vi "EditorPopUp.vi"(8 "error in (no error)":errorcluster, 11 "MAUI.Editor":refnum<class "MAUI.Editor.lvclass">) -> (0 "error out":errorcluster, 3 "MAUI.Editor out":refnum<class "MAUI.Editor.lvclass">)   [LabVIEW 2020, in "MAUI.Editor.lvclass"]
uses:
  MAUI.Editor/MAUI.Editor.lvclass
panel:
  in  "Listbox":i32(listbox)
  in  "Save":bool
  in  "Select":bool
  in  "Refresh":bool
  in  "Configure":bool
  in  "New":bool
  in  "Delete":bool
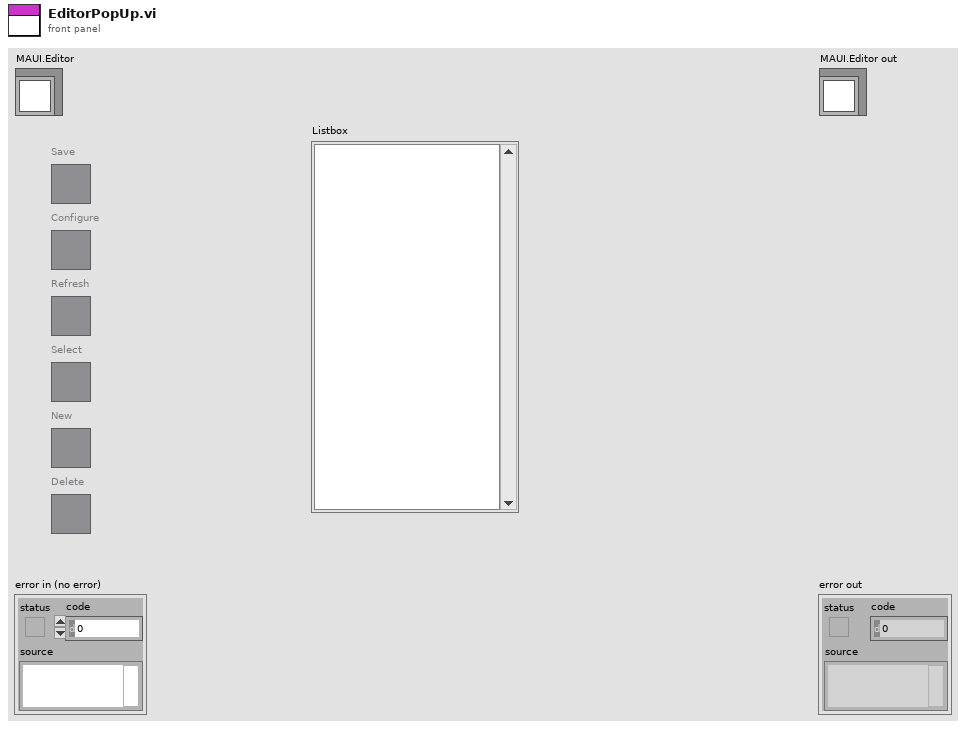
[diagram p1: front panel]
types:
  T1 = enum32{"Invalid", "Standard", "Closed", "Hidden", "Minimized", "Maximized"}
  T2 = enum32{"invalid app kind", "Development System", "Run Time System", "Student Edition", "Embedded LabVIEW", "Evaluation", "Custom"}
  T3 = cluster{"Core":cluster{"Current VI Reference":refnum<vi>, "Close Panel on Exit?":bool}, "MAUI.Editor":refnum<class "MAUI.Editor.lvclass">}
  T4 = cluster{"Current VI Reference":refnum<vi>, "Close Panel on Exit?":bool}
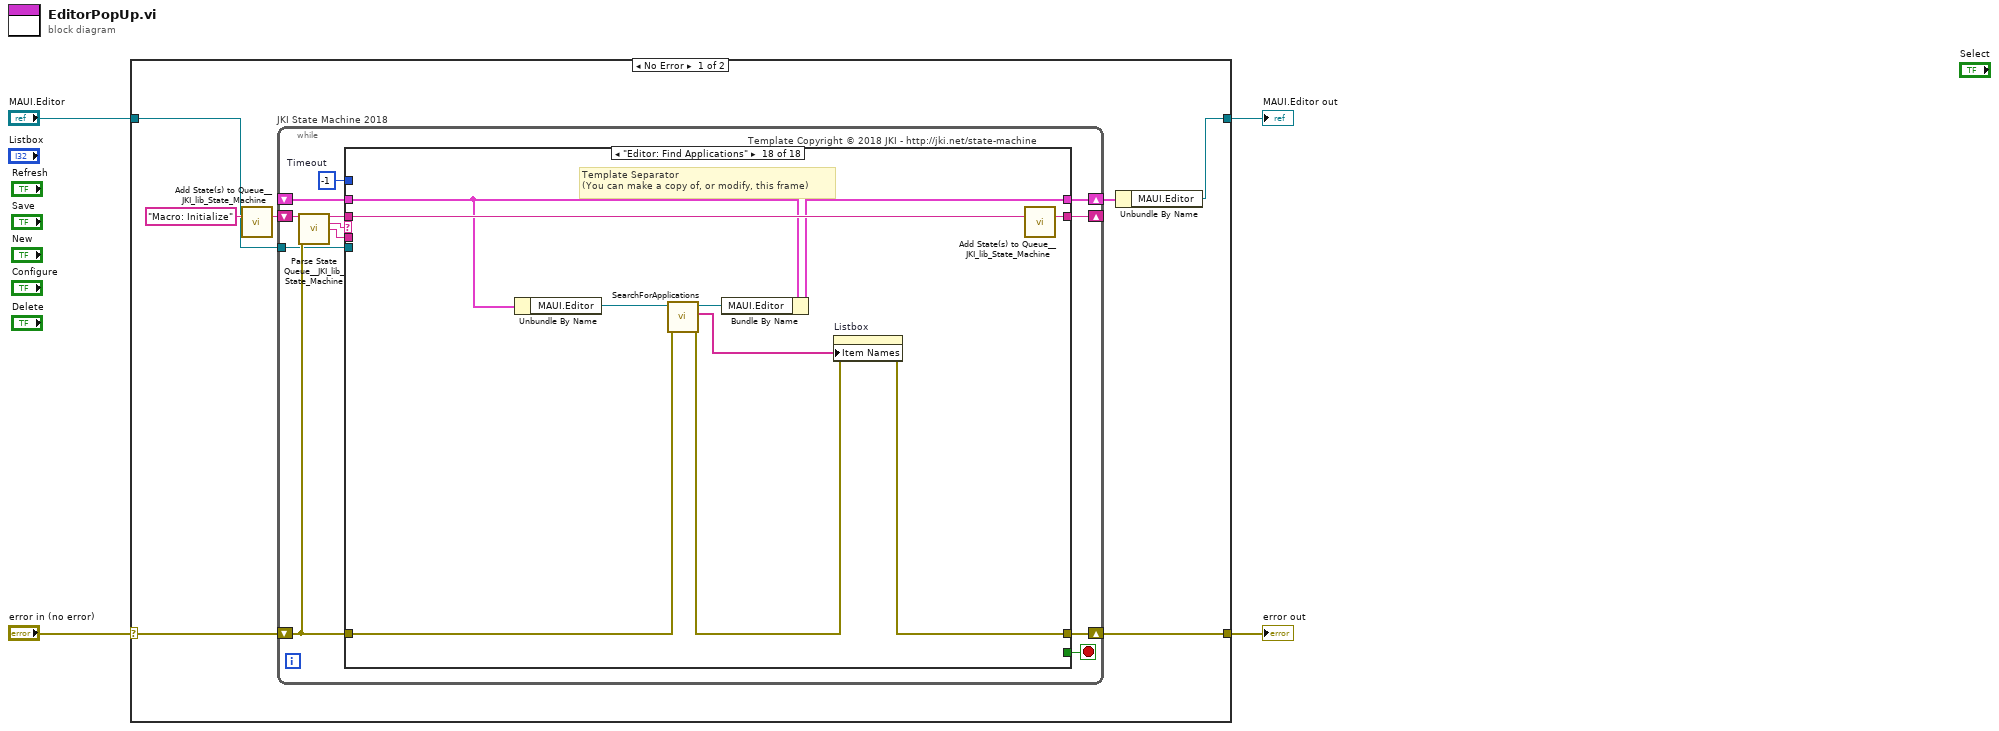
[diagram p0: block diagram]
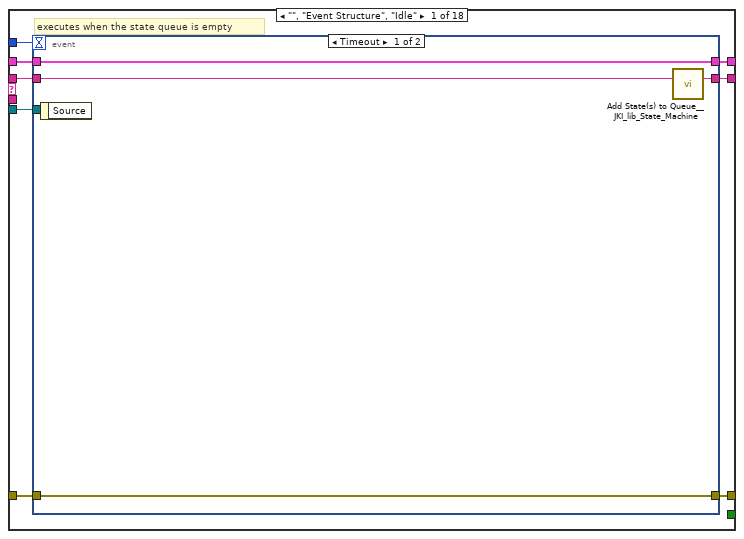
[diagram p2: hidden frame]
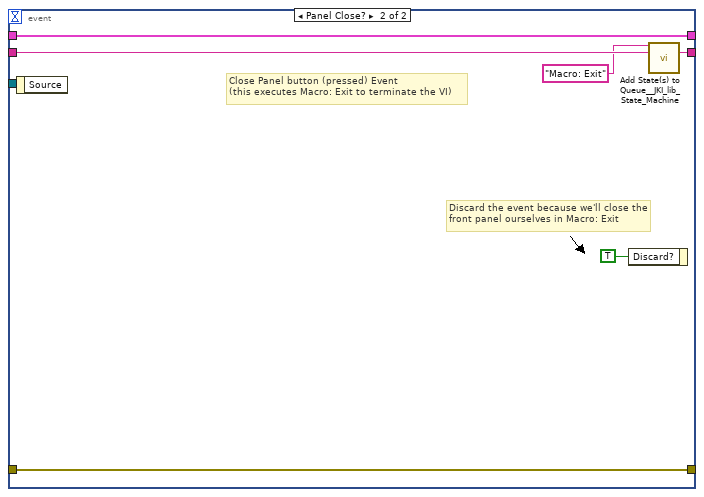
[diagram p3: hidden frame]
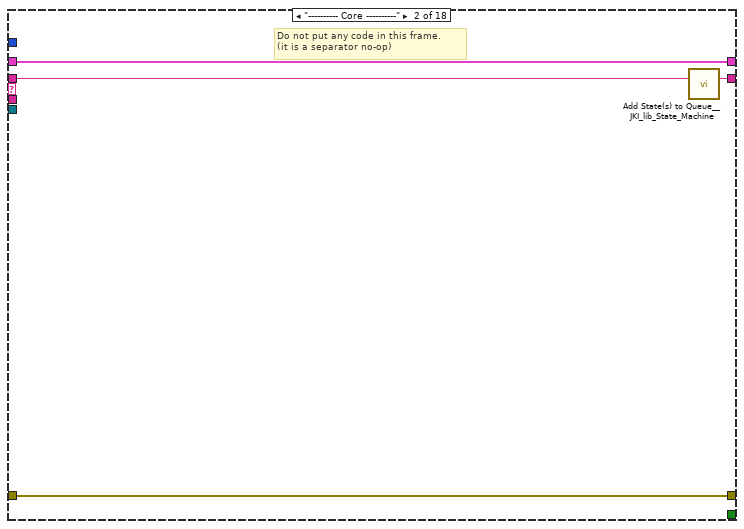
[diagram p4: hidden frame]
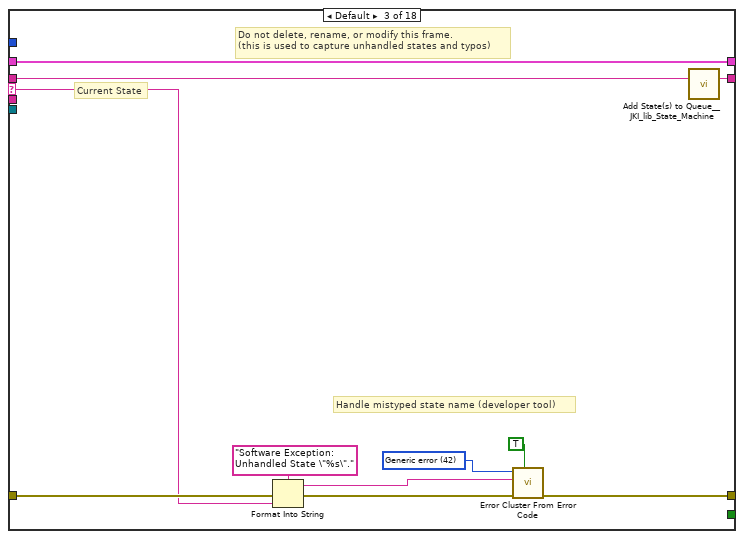
[diagram p5: hidden frame]
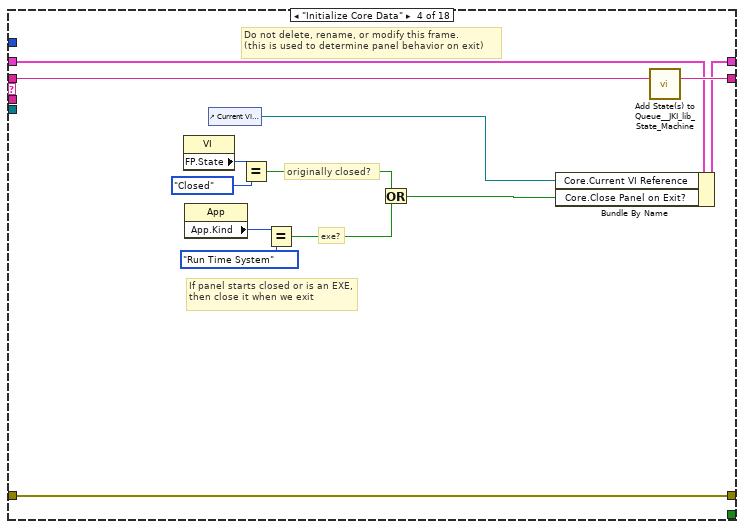
[diagram p6: hidden frame]
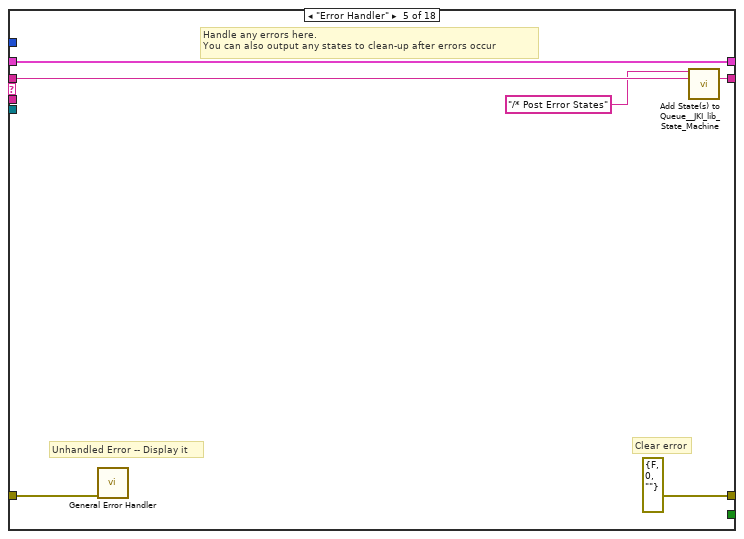
[diagram p7: hidden frame]
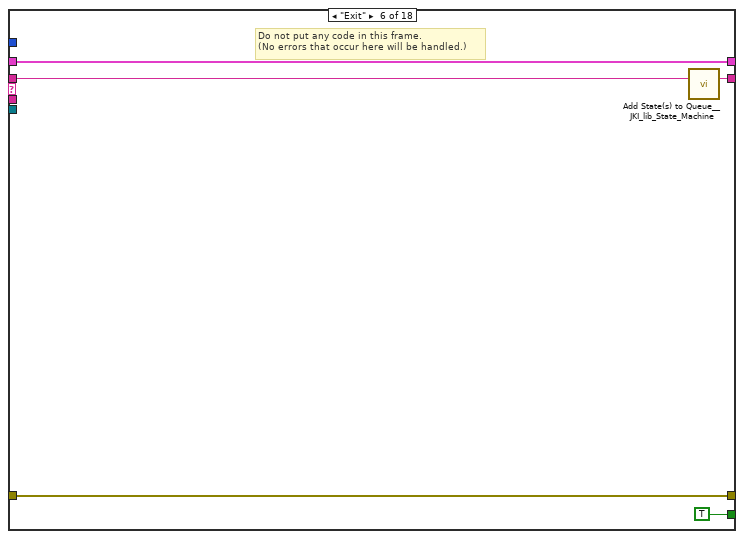
[diagram p8: hidden frame]
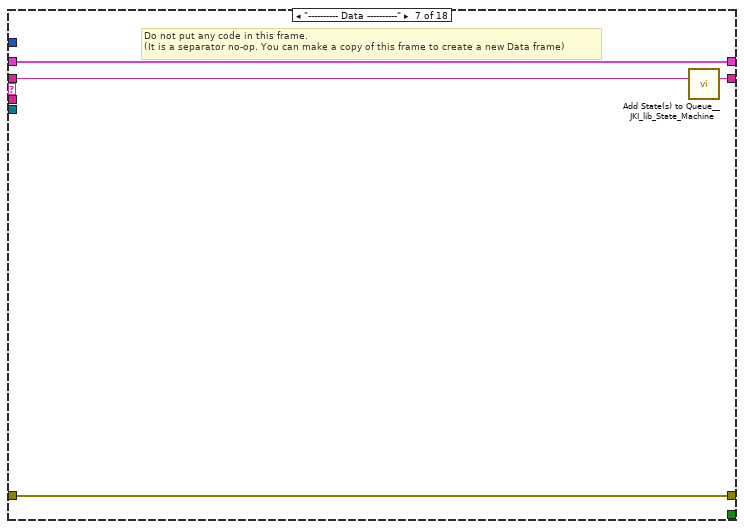
[diagram p9: hidden frame]
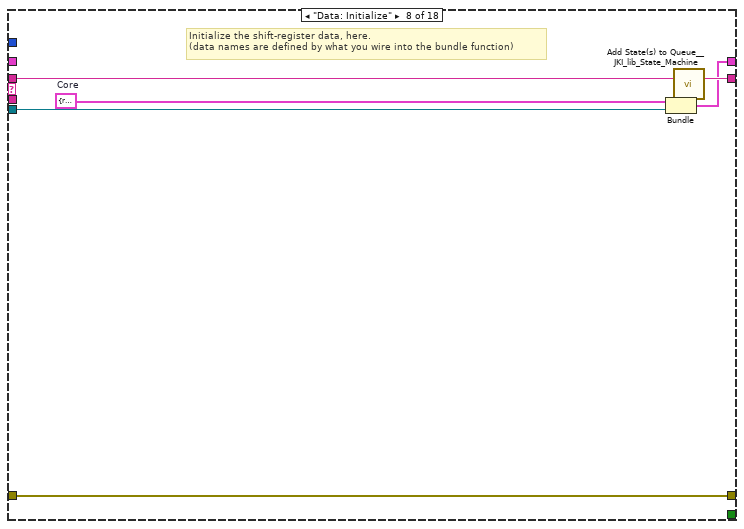
[diagram p10: hidden frame]
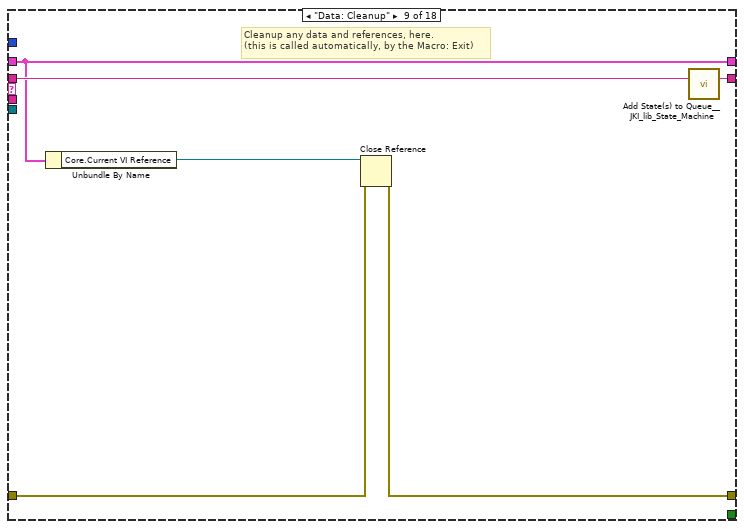
[diagram p11: hidden frame]
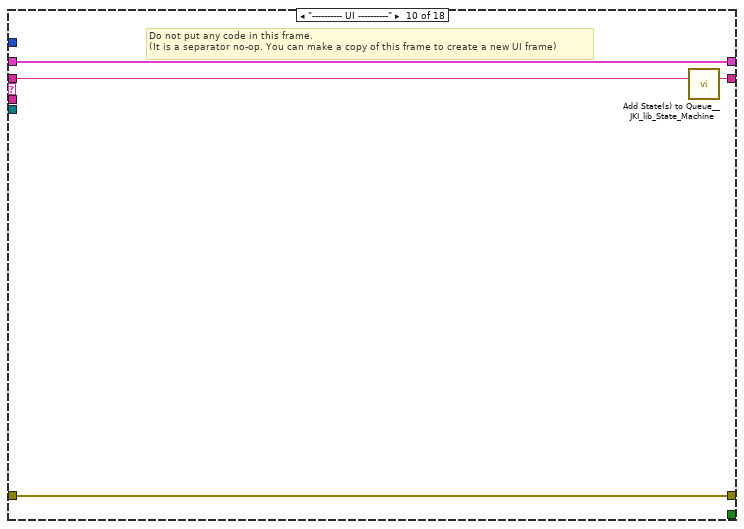
[diagram p12: hidden frame]
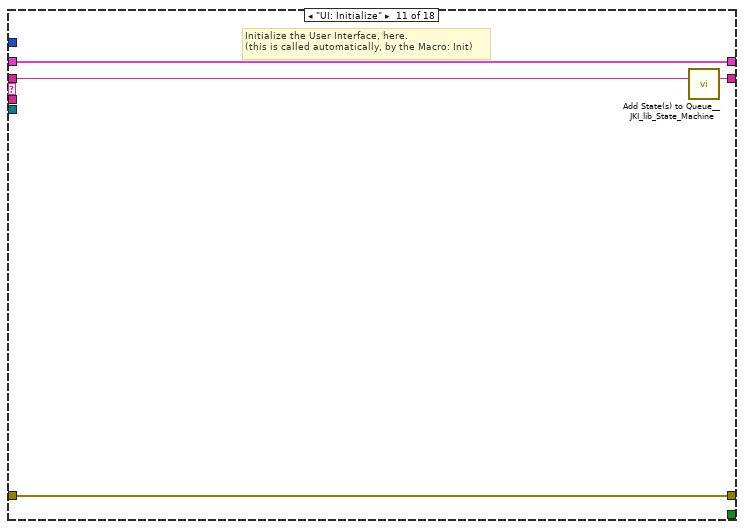
[diagram p13: hidden frame]
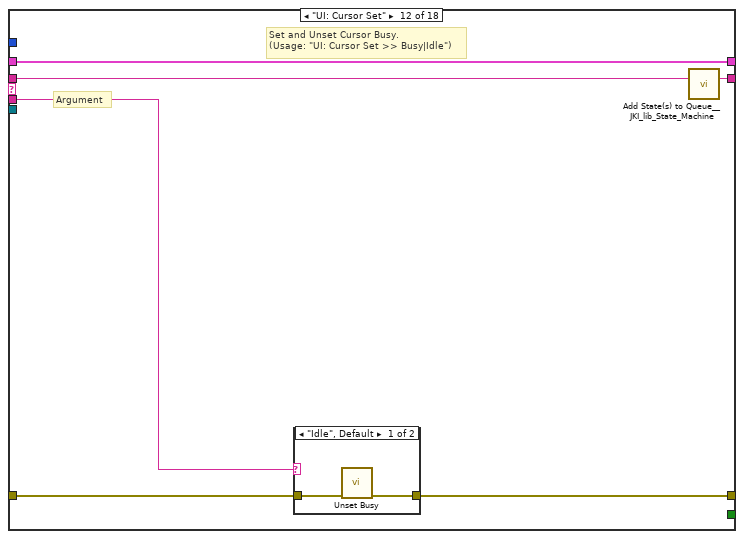
[diagram p14: hidden frame]
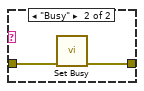
[diagram p15: hidden frame]
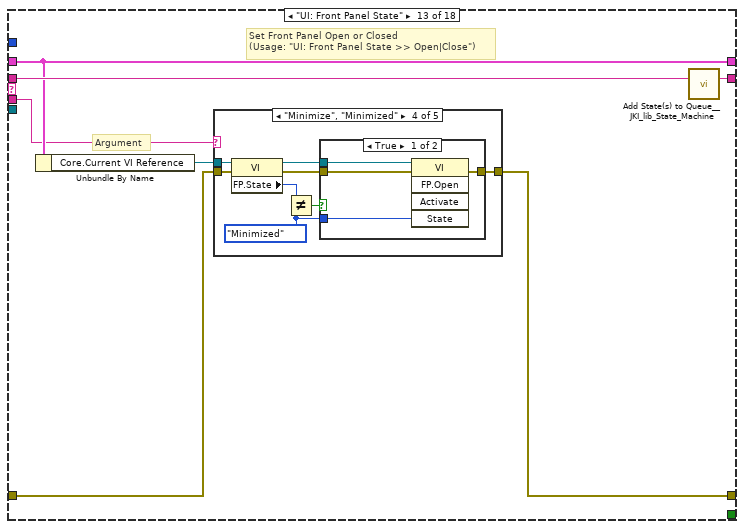
[diagram p16: hidden frame]
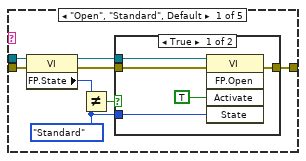
[diagram p17: hidden frame]
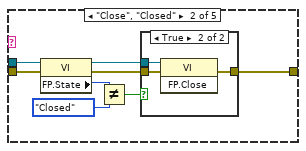
[diagram p19: hidden frame]
diagram:
  n1 = case shown="No Error" "error in (no error)" {
    selector: "error in (no error)" -> [w5 w223]
    tunnel: [w6 w223] -> w3
    tunnel: [w7 w222] -> w1
    tunnel: "MAUI.Editor" -> [w8 w222]
    frame No Error {
      n2 = call <vilib>:"Add State(s) to Queue__JKI_lib_State_Machine.vi"("State(s) in (\"\")"="Macro: Initialize") -> ("States Out"=w11:string)  [unwired: 14 in]
      n3 = while "JKI State Machine 2018" {
        shift-right: [w16] -> w9
        shift-left: _ -> [w15]
        shift-right: [w19] -> w6
        shift-left: w5 -> [w13]
        shift-right: [w18] -> _
        shift-left: w11 -> [w20]
        tunnel: w8 -> [w12]
        stop <- w17 stop-if-true
        w14 = -1  # Timeout
        # "Template Copyright © 2018 JKI - http://jki.net/state-machine"
        n4 = call <vilib>:"Parse State Queue__JKI_lib_State_Machine.vi"("State Queue"=w20, "Error In (no error)"=w13) -> ("Remaining States"=w22:string, "Current State"=w23:string, "Arguments"=w21:string)  [unwired: 11 in]
        n5 = case shown="\"Editor: Find Applications\"" w23 {
          selector: w23 -> [_ _ w46 _ _ _ _ _ _ _ _ _ _ _ _ _ _ _]
          tunnel: w22 -> [w31 w45 w50 w69 w75 w80 w84 w90 w96 w100 w104 w110 w121 w190 w195 w205 w211 w221]
          tunnel: w21 -> [_ _ _ _ _ _ _ _ _ _ _ w105 w115 _ _ _ _ _]
          tunnel: w15 -> [w29 w42 w48 w62 w72 w78 w81 _ w91 w97 w102 w108 w117 w187 w192 w202 w207 w217]
          tunnel: [w28 w43 w52 w66 errorcluster {"status"=FALSE, "code"=0, "source"=""} ("error out") w77 w82 w87 w92 w98 w101 w106 w118 w188 w193 w203 w209 w212] -> w19
          tunnel: w13 -> [w27 w43 w51 w66 w71 w77 w82 w87 w93 w98 w101 w107 w119 w188 w193 w203 w209 w215]
          tunnel: [w30 w44 w49 w68 w74 w79 w83 w89 w95 w99 w103 w109 w120 w189 w194 w204 w210 w220] -> w18
          tunnel: [_ _ _ _ _ TRUE _ _ _ _ _ _ _ _ _ _ _ _] -> w17
          tunnel: [w26 w42 w48 w67 w72 w78 w81 w88 w91 w97 w102 w108 w117 w187 w192 w202 w208 w218] -> w16
          tunnel: w14 -> [w25 _ _ _ _ _ _ _ _ _ _ _ _ _ _ _ _ _]
          tunnel: w12 -> [w24 _ _ _ _ _ _ w85 _ _ _ _ _ _ _ _ _ _]
          frame "", "Event Structure", "Idle" {
            # "executes when the state queue is empty"
            n6 = event shown="[0] Timeout" {
              selector: _ -> [_ _]
              dyn-events: _ -> [_ _]
              timeout: w25 -> [_ _]
              tunnel: w31 -> [w35 w41]
              tunnel: [w34 w40] -> w30
              tunnel: w29 -> [w32 w38]
              tunnel: [w33 w39] -> w28
              tunnel: w27 -> [w33 w39]
              tunnel: [w32 w38] -> w26
              tunnel: w24 -> [_ _]
              event Timeout {
                n7 = event-data() -> ()  [unwired: 1 in, 1 out]
                n8 = call <vilib>:"Add State(s) to Queue__JKI_lib_State_Machine.vi"("State(s) in (\"\")"=w35) -> ("States Out"=w34:string)  [unwired: 14 in]
              }
              event Panel Close? {
                # "Discard the event because we'll close the front panel ourselves in Macro: Exit"
                # "Close Panel button (pressed) Event\n(this executes Macro: Exit to terminate the VI)"
                n9 = event-data() -> ()  [unwired: 1 in, 1 out]
                n10 = event-data("Discard?"=TRUE) -> ()  [unwired: 1 in, 1 out]
                n11 = call <vilib>:"Add State(s) to Queue__JKI_lib_State_Machine.vi"("State(s) in Front (\"\")"="Macro: Exit", "State(s) in (\"\")"=w41) -> ("States Out"=w40:string)  [unwired: 13 in]
              }
            }
          }
          frame "---------- Core ----------" {
            # "Do not put any code in this frame.\n(it is a separator no-op)"
            n12 = call <vilib>:"Add State(s) to Queue__JKI_lib_State_Machine.vi"("State(s) in (\"\")"=w45) -> ("States Out"=w44:string)  [unwired: 14 in]
          }
          frame Default {
            w55 = 42 items=["No error", "Argument error", "Memory is full", "Out of zone", "End of file", "File already open", "Generic file I/O error", "File not found", "File permission error", "Disk is full", "Duplicate path", "Too many files open", "System feature not enabled", "Resource file not found", "Cannot add resource", "Resource not found", "Image not found", "Image memory error", "Pen does not exist", "Config type invalid", "Config token not found", "Config parse error", "Config memory error", "Bad external code format", "Bad external code offset", "External code not present", "Null window", "Destroy window error", "Null menu", "Print aborted", "Bad print record", "Print driver error", "Windows error during printing", "Memory error during printing", "Print dialog error", "Generic print error", "Invalid device refnum", "Device not found", "Device parameter error", "Device unit error", "Cannot open device", "Device call aborted", "Generic error", "Cancelled by user", "Object ID too low", "Object ID too high", "Object not in heap", "Unknown heap", "Unknown object (invalid DefProc)", "Unknown object (DefProc not in table)", "Message out of range", "Invalid (null) method", "Unknown message", "Manager call not supported", "Bad address", "Network operation in progress", "Network operation timed out", "Connection is busy", "Network attribute not supported", "Network error", "Address in use", "System out of memory", "Connection aborted", "Connection refused", "Not connected", "Already connected", "Connection closed", "Initialization error (interapplication manager)", "Bad occurrence", "Wait on unbound occurrence handler", "Occurrence queue overflow", "Datalog type conflict", "Unused", "Unrecognized type (interapplication manager)", "Memory corrupt", "Failed to make temporary DLL", "Old CIN version", "Drag socket not found", "Failed to load drop-object", "Failed to register OLE object", "Failed to release OLE object", "Format specifier type mismatch", "Unknown format specifier", "Too few format specifiers", "Too many format specifiers", "Scan failed", "Newer CIN version", "Error converting to variant", "Runtime menu error", "Password tampered", "Variant attribute not found", "Incompatible variant data type", "Event data is not available", "Event Store is not present", "Occurrence is not found", "Event Queue is not created", "Event info is not available", "Refnum passed is NULL", "Error retrieving Class GUID", "Error retrieving CoClass GUID", "Error retrieving TypeLib GUID.", "Bad built application magic bytes.", "Specific driver is different from the specific driver associated with the Logical Name.", "There is no session opened to the class driver.", "Max Error", "MAX - Error with config objects", "MAX - Error loading configuration", "MAX - Group not supported"]
            # "Current State"
            # "Do not delete, rename, or modify this frame.\n(this is used to capture unhandled states and typos)"
            # "Handle mistyped state name (developer tool)"
            n13 = Format Into String(format string="Software Exception: Unhandled State \"%s\"." ("message"), error in=w51, w46) -> (resulting string=w54:string, error out=w53:errorcluster)  [unwired: 1 in]
            n14 = call <vilib>:"Error Cluster From Error Code.vi"("show call chain? (False)"=TRUE, "error in (no error)"=w53, "error message (\"\")"=w54, "error code (0)"=w55) -> ("error out"=w52:errorcluster)  [unwired: 5 in]
            n15 = call <vilib>:"Add State(s) to Queue__JKI_lib_State_Machine.vi"("State(s) in (\"\")"=w50) -> ("States Out"=w49:string)  [unwired: 14 in]
          }
          frame "Initialize Core Data" {
            # "Do not delete, rename, or modify this frame.\n(this is used to determine panel behavior on exit)"
            # "originally closed?"
            # "exe?"
            # "If panel starts closed or is an EXE, then close it when we exit"
            n16 = property class="VI"() -> ("FP.State"=w59:T1)  [unwired: 2 in, 2 out]
            n17 = property class="App"() -> ("App.Kind"=w65:T2)  [unwired: 2 in, 2 out]
            n18 = control-ref of="Current VI Reference"() -> (w60:refnum<vi>)
            n19 = Equal?(x=w59, y=T1."Closed" ("Front Panel Window:State")) -> (x = y?=w57:bool)
            n20 = Equal?(x=w65, y=T2."Run Time System" ("Application:Kind")) -> (x = y?=w63:bool)
            n21 = Or(x=w57, y=w63) -> (x .or. y?=w61:bool)
            n22 = Bundle By Name(cluster=w62, "Core.Current VI Reference"=w60, "Core.Close Panel on Exit?"=w61) -> (w67:T3)
            n23 = call <vilib>:"Add State(s) to Queue__JKI_lib_State_Machine.vi"("State(s) in (\"\")"=w69) -> ("States Out"=w68:string)  [unwired: 14 in]
          }
          frame "Error Handler" {
            # "Unhandled Error -- Display it"
            # "Handle any errors here.\nYou can also output any states to clean-up after errors occur"
            # "Clear error"
            n24 = call <vilib>:"General Error Handler.vi"("error in (no error)"=w71) -> ()  [unwired: 10 in, 5 out]
            n25 = call <vilib>:"Add State(s) to Queue__JKI_lib_State_Machine.vi"("State(s) in Front (\"\")"="/* Post Error States", "State(s) in (\"\")"=w75) -> ("States Out"=w74:string)  [unwired: 13 in]
          }
          frame "Exit" {
            # "Do not put any code in this frame.\n(No errors that occur here will be handled.)"
            n26 = call <vilib>:"Add State(s) to Queue__JKI_lib_State_Machine.vi"("State(s) in (\"\")"=w80) -> ("States Out"=w79:string)  [unwired: 14 in]
          }
          frame "---------- Data ----------" {
            # "Do not put any code in this frame.\n(It is a separator no-op. You can make a copy of this frame to create a new Data frame)"
            n27 = call <vilib>:"Add State(s) to Queue__JKI_lib_State_Machine.vi"("State(s) in (\"\")"=w84) -> ("States Out"=w83:string)  [unwired: 14 in]
          }
          frame "Data: Initialize" {
            w86 = T4 {"Current VI Reference"=refnum, "Close Panel on Exit?"=FALSE}  # Core
            # "Initialize the shift-register data, here.\n(data names are defined by what you wire into the bundle function)"
            n28 = Bundle("Core"=w86, "MAUI.Editor"=w85) -> (w88:T3)  [unwired: 1 in]
            n29 = call <vilib>:"Add State(s) to Queue__JKI_lib_State_Machine.vi"("State(s) in (\"\")"=w90) -> ("States Out"=w89:string)  [unwired: 14 in]
          }
          frame "Data: Cleanup" {
            # "Cleanup any data and references, here.\n(this is called automatically, by the Macro: Exit)"
            n30 = Unbundle By Name(w91) -> ("Core.Current VI Reference"=w94:refnum<vi>)
            n31 = Close Reference(reference=w94, error in (no error)=w93) -> (error out=w92:errorcluster)
            n32 = call <vilib>:"Add State(s) to Queue__JKI_lib_State_Machine.vi"("State(s) in (\"\")"=w96) -> ("States Out"=w95:string)  [unwired: 14 in]
          }
          frame "---------- UI ----------" {
            # "Do not put any code in this frame.\n(It is a separator no-op. You can make a copy of this frame to create a new UI frame)"
            n33 = call <vilib>:"Add State(s) to Queue__JKI_lib_State_Machine.vi"("State(s) in (\"\")"=w100) -> ("States Out"=w99:string)  [unwired: 14 in]
          }
          frame "UI: Initialize" {
            # "Initialize the User Interface, here.\n(this is called automatically, by the Macro: Init)"
            n34 = call <vilib>:"Add State(s) to Queue__JKI_lib_State_Machine.vi"("State(s) in (\"\")"=w104) -> ("States Out"=w103:string)  [unwired: 14 in]
          }
          frame "UI: Cursor Set" {
            # "Argument"
            # "Set and Unset Cursor Busy.\n(Usage: \"UI: Cursor Set >> Busy|Idle\")"
            n35 = case shown="\"Idle\", Default" w105 {
              tunnel: w107 -> [w112 w114]
              tunnel: [w111 w113] -> w106
              frame "Idle", Default {
                n36 = call <vilib>:"Unset Busy.vi"("error in (no error)"=w112) -> ("error out"=w111:errorcluster)  [unwired: 10 in]
              }
              frame "Busy" {
                n37 = call <vilib>:"Set Busy.vi"("error in (no error)"=w114) -> ("error out"=w113:errorcluster)  [unwired: 9 in, 1 out]
              }
            }
            n38 = call <vilib>:"Add State(s) to Queue__JKI_lib_State_Machine.vi"("State(s) in (\"\")"=w110) -> ("States Out"=w109:string)  [unwired: 14 in]
          }
          frame "UI: Front Panel State" {
            # "Argument"
            # "Set Front Panel Open or Closed\n(Usage: \"UI: Front Panel State >> Open|Close\")"
            n39 = Unbundle By Name(w117) -> ("Core.Current VI Reference"=w116:refnum<vi>)
            n40 = case shown="\"Minimize\", \"Minimized\"" w115 {
              tunnel: w119 -> [w127 w142 w153 w166 w179]
              tunnel: [w129 w143 w155 w168 w181] -> w118
              tunnel: w116 -> [w128 w140 w154 w167 w180]
              frame "Open", "Standard", Default {
                w122 = T1."Standard" ("State")
                n41 = property class="VI"(reference=w128, error in=w127) -> (reference out=w125:refnum<vi>, error out=w126:errorcluster, "FP.State"=w124:T1)
                n42 = Not Equal?(x=w124, y=w122) -> (x != y?=w123:bool)
                n43 = case shown="True" w123 {
                  tunnel: [w133 w135] -> w129
                  tunnel: w126 -> [w132 w135]
                  tunnel: w125 -> [w131 _]
                  tunnel: w122 -> [w130 _]
                  frame True {
                    n44 = invoke class="VI" method="FP.Open"(reference=w131, error in=w132, "Activate"=TRUE, "State"=w130) -> (error out=w133:errorcluster)  [unwired: 1 in, 4 out]
                  }
                  frame False {
                  }
                }
              }
              frame "Close", "Closed" {
                n45 = property class="VI"(reference=w140, error in=w142) -> (reference out=w139:refnum<vi>, error out=w141:errorcluster, "FP.State"=w137:T1)
                n46 = Not Equal?(x=w137, y=T1."Closed" ("Front Panel Window:State")) -> (x != y?=w136:bool)
                n47 = case shown="True" w136 {
                  tunnel: [w144 w147] -> w143
                  tunnel: w141 -> [w144 w146]
                  tunnel: w139 -> [_ w145]
                  frame False {
                  }
                  frame True {
                    n48 = invoke class="VI" method="FP.Close"(reference=w145, error in=w146) -> (error out=w147:errorcluster)  [unwired: 1 in, 2 out]
                  }
                }
              }
              frame "Hidden", "Hide" {
                w148 = T1."Hidden" ("State")
                n49 = property class="VI"(reference=w154, error in=w153) -> (reference out=w151:refnum<vi>, error out=w152:errorcluster, "FP.State"=w150:T1)
                n50 = Not Equal?(x=w150, y=w148) -> (x != y?=w149:bool)
                n51 = case shown="True" w149 {
                  tunnel: [w159 w160] -> w155
                  tunnel: w152 -> [w158 w160]
                  tunnel: w151 -> [w157 _]
                  tunnel: w148 -> [w156 _]
                  frame True {
                    n52 = invoke class="VI" method="FP.Open"(reference=w157, error in=w158, "State"=w156) -> (error out=w159:errorcluster)  [unwired: 2 in, 4 out]
                  }
                  frame False {
                  }
                }
              }
              frame "Minimize", "Minimized" {
                w161 = T1."Minimized" ("State")
                n53 = property class="VI"(reference=w167, error in=w166) -> (reference out=w164:refnum<vi>, error out=w165:errorcluster, "FP.State"=w163:T1)
                n54 = Not Equal?(x=w163, y=w161) -> (x != y?=w162:bool)
                n55 = case shown="True" w162 {
                  tunnel: [w172 w173] -> w168
                  tunnel: w165 -> [w171 w173]
                  tunnel: w164 -> [w170 _]
                  tunnel: w161 -> [w169 _]
                  frame True {
                    n56 = invoke class="VI" method="FP.Open"(reference=w170, error in=w171, "State"=w169) -> (error out=w172:errorcluster)  [unwired: 2 in, 4 out]
                  }
                  frame False {
                  }
                }
              }
              frame "Maximize", "Maximized" {
                w174 = T1."Maximized" ("State")
                n57 = property class="VI"(reference=w180, error in=w179) -> (reference out=w177:refnum<vi>, error out=w178:errorcluster, "FP.State"=w176:T1)
                n58 = Not Equal?(x=w176, y=w174) -> (x != y?=w175:bool)
                n59 = case shown="True" w175 {
                  tunnel: [w185 w186] -> w181
                  tunnel: w178 -> [w184 w186]
                  tunnel: w177 -> [w183 _]
                  tunnel: w174 -> [w182 _]
                  frame True {
                    n60 = invoke class="VI" method="FP.Open"(reference=w183, error in=w184, "State"=w182) -> (error out=w185:errorcluster)  [unwired: 2 in, 4 out]
                  }
                  frame False {
                  }
                }
              }
            }
            n61 = call <vilib>:"Add State(s) to Queue__JKI_lib_State_Machine.vi"("State(s) in (\"\")"=w121) -> ("States Out"=w120:string)  [unwired: 14 in]
          }
          frame "---------- Macro ----------" {
            # "Do not put any code in this frame.\n(It is a separator no-op. You can make a copy of this frame to create a new Macro frame)"
            n62 = call <vilib>:"Add State(s) to Queue__JKI_lib_State_Machine.vi"("State(s) in (\"\")"=w190) -> ("States Out"=w189:string)  [unwired: 14 in]
          }
          frame "Macro: Initialize" {
            w191 = "Data: Initialize\nInitialize Core Data\nUI: Initialize\nUI: Front Panel State >> Open"  # Data: Initialize Initialize Core Data UI: Initialize UI: Front Panel State >> Open
            # "Initialization Macro\n(This is called once, when the VI starts)"
            n63 = call <vilib>:"Add State(s) to Queue__JKI_lib_State_Machine.vi"("State(s) in Front (\"\")"=w191, "State(s) in (\"\")"=w195) -> ("States Out"=w194:string)  [unwired: 13 in]
          }
          frame "Macro: Exit" {
            # "Exit Macro\n(This is called once, when the VI exits)"
            n64 = Unbundle By Name(w202) -> ("Core.Close Panel on Exit?"=w201:bool)
            n65 = Select(t="UI: Front Panel State >> Close", s=w201, f="") -> (s? t:f=w198:string)
            n66 = call <vilib>:"Add State(s) to Queue__JKI_lib_State_Machine.vi"("State(s) in (\"\")"=w198, "State(s) at Back (\"\")"="Data: Cleanup\nExit") -> ("States Out"=w196:string)  [unwired: 13 in]
            n67 = call <vilib>:"Add State(s) to Queue__JKI_lib_State_Machine.vi"("State(s) in Front (\"\")"=w196, "State(s) in (\"\")"=w205) -> ("States Out"=w204:string)  [unwired: 13 in]
          }
          frame "---------- Editor ----------" {
            # "Template Separator\n(You can make a copy of, or modify, this frame)"
            n68 = Unbundle By Name(w207) -> ("MAUI.Editor"=w206:refnum<class "MAUI.Editor.lvclass">)
            n69 = Bundle By Name(cluster=w207, "MAUI.Editor"=w206) -> (w208:T3)
            n70 = call <vilib>:"Add State(s) to Queue__JKI_lib_State_Machine.vi"("State(s) in (\"\")"=w211) -> ("States Out"=w210:string)  [unwired: 14 in]
          }
          frame "Editor: Find Applications" {
            # "Template Separator\n(You can make a copy of, or modify, this frame)"
            n71 = Unbundle By Name(w217) -> ("MAUI.Editor"=w219:refnum<class "MAUI.Editor.lvclass">)
            n72 = call "SearchForApplications.vi"("error in (no error)"=w215, "MAUI.Editor in"=w219) -> ("error out"=w213:errorcluster, "folder names"=w214:string[], "MAUI.Editor out"=w216:refnum<class "MAUI.Editor.lvclass">)  [unwired: 7 in]
            n73 = Bundle By Name(cluster=w217, "MAUI.Editor"=w216) -> (w218:T3)
            n74 = property on="Listbox" class="LstBox (strict)"(error in=w213, "Item Names"=w214) -> (error out=w212:errorcluster)  [unwired: 1 in, 1 out]
            n75 = call <vilib>:"Add State(s) to Queue__JKI_lib_State_Machine.vi"("State(s) in (\"\")"=w221) -> ("States Out"=w220:string)  [unwired: 14 in]
          }
        }
      }
      n76 = Unbundle By Name(w9) -> ("MAUI.Editor"=w7:refnum<class "MAUI.Editor.lvclass">)
    }
    frame Error {
    }
  }
  "error out" <- w3
  "MAUI.Editor out" <- w1
